vi "流水灯.vi"() -> ()   [LabVIEW 2017]
panel:
  in  "停止 2":bool
  in  "滑动杆":dbl(slide) scale=0.0..500.0
  out "布尔":bool
  out "布尔 2":bool
  out "布尔 3":bool
  out "布尔 4":bool
  out "布尔 5":bool
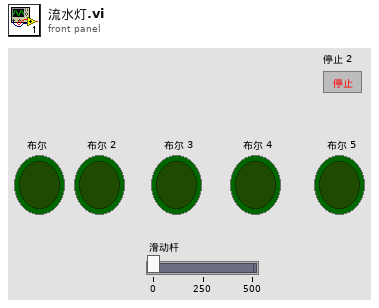
[diagram p1: front panel]
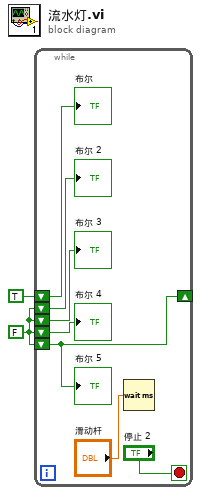
[diagram p0: block diagram]
diagram:
  w1 = FALSE
  n1 = while {
    shift-right: [w3] -> _
    shift-left: TRUE -> [w7]
    shift-left: w1 -> [w6]
    shift-left: w1 -> [w5]
    shift-left: w1 -> [w4]
    shift-left: w1 -> [w3]
    stop <- "停止 2" stop-if-true
    n2 = Wait (ms)(milliseconds to wait="滑动杆") -> ()  [unwired: 1 out]
    "布尔" <- w7
    "布尔 2" <- w6
    "布尔 3" <- w5
    "布尔 4" <- w4
    "布尔 5" <- w3
  }
